vi "INI.GetSettings.vi"(8 "error in (no error)":errorcluster, 11 "INI Folder Location":path) -> (0 "error out":errorcluster, 3 "INI.Settings":T1={"Build Location"=path "C:/Simple Sequence Editor/SequenceRepo", "LoggingLocation"=path ""})   [LabVIEW 2013, in "Simple Sequence Tools - Shared.lvlib"]
uses:
  Simple Sequence Tools - Shared.lvlib
  Types/INI.Settings
  Main.Constants.vi
  <vilib>/Utility/config.llb/Read Key (Path).vi
  <vilib>/Utility/config.llb/Write Key (Path).vi
  <vilib>/Utility/config.llb/NI_LVConfig.lvlib
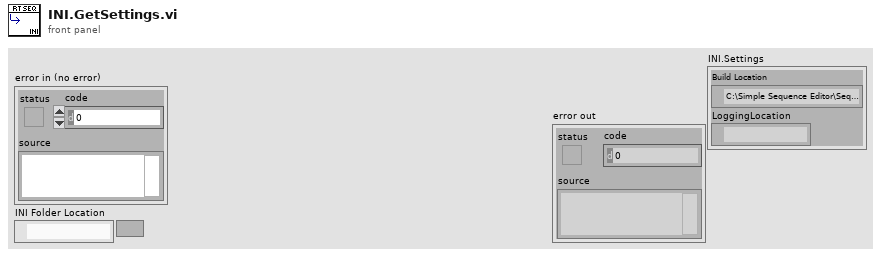
[diagram p1: front panel]
types:
  T1 = typedef "Simple Sequence Tools - Shared.lvlib/INI.Settings" = cluster{"Build Location":path, "LoggingLocation":path}
  T2 = typedef "NI_LVConfig.lvlib/Config Data RefNum.ctl" = refnum<k1>
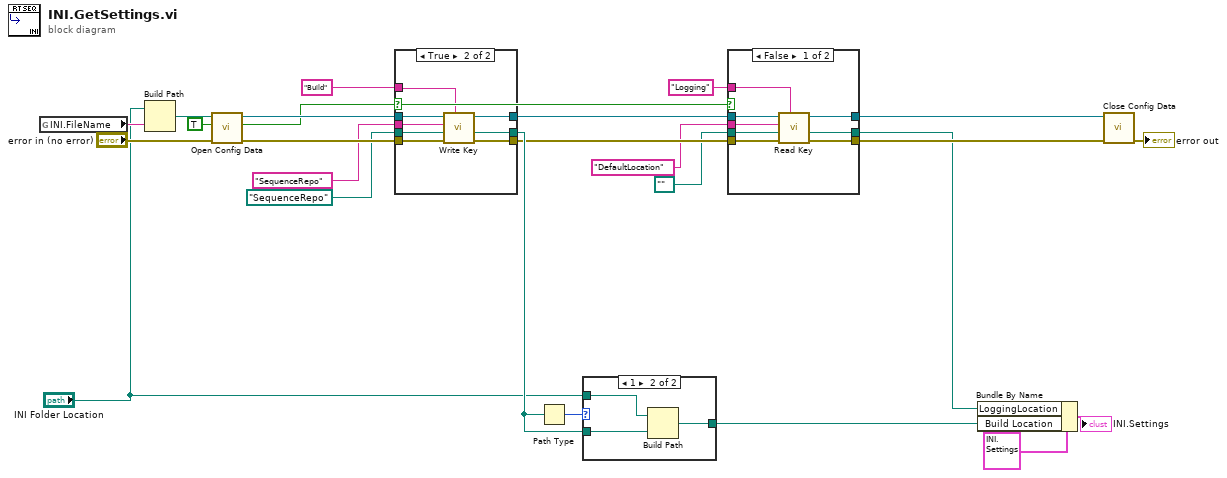
[diagram p0: block diagram]
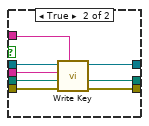
[diagram p2: hidden frame]
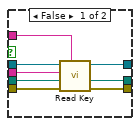
[diagram p3: hidden frame]
diagram:
  n1 = global read "Main.Constants.vi" "INI.FileName"() -> (w17:string)
  n2 = Build Path(base path="INI Folder Location", name or relative path=w17) -> (appended path=w18:path)
  n3 = call <vilib>:"Open Config Data.vi"("error in (no error)"="error in (no error)", "create file if necessary (T)"=TRUE, "configuration file path"=w18) -> ("error out"=w24:errorcluster, "file created?"=w8:bool, "refnum"=w25:T2)  [unwired: 6 in]
  n4 = case shown="True" w8 {
    tunnel: w25 -> [w33 w38]
    tunnel: w24 -> [w32 w40]
    tunnel: [w31 w36] -> w10
    tunnel: [w30 w34] -> w5
    tunnel: "Build" ("section") -> [w29 w37]
    tunnel: "SequenceRepo" ("key") -> [w28 w39]
    tunnel: path "SequenceRepo" ("default value") -> [w27 w35]
    tunnel: [w26 w35] -> w19
    frame False {
      n5 = call-poly <vilib>:"Read Key.vi"("section"=w29, "error in (no error)"=w32, "default value"=w27, "key"=w28, "refnum"=w33) -> ("error out"=w31:errorcluster, "value"=w26:path, "refnum out"=w30:T2)  [unwired: 3 in, 1 out]
    }
    frame True {
      n6 = call-poly <vilib>:"Write Key.vi"("section"=w37, "error in (no error)"=w40, "value"=w35, "key"=w39, "refnum"=w38) -> ("error out"=w36:errorcluster, "refnum out"=w34:T2)  [unwired: 4 in, 1 out]
    }
  }
  n7 = Path Type(1:w19) -> (0:w20:i16)
  n8 = case shown="1" w20 {
    tunnel: w19 -> [w41 w44]
    tunnel: [w41 w43] -> w12
    tunnel: "INI Folder Location" -> [_ w42]
    frame 0, Default {
    }
    frame 1 {
      n9 = Build Path(base path=w42, name or relative path=w44) -> (appended path=w43:path)
    }
  }
  n10 = case shown="False" w8 {
    tunnel: w5 -> [w52 w57]
    tunnel: w10 -> [w51 w59]
    tunnel: [w50 w55] -> w9
    tunnel: [w49 w53] -> w4
    tunnel: "Logging" ("section") -> [w48 w56]
    tunnel: "DefaultLocation" ("key") -> [w47 w58]
    tunnel: path "" ("default value") -> [w46 w54]
    tunnel: [w45 w54] -> w2
    frame False {
      n11 = call-poly <vilib>:"Read Key.vi"("section"=w48, "error in (no error)"=w51, "default value"=w46, "key"=w47, "refnum"=w52) -> ("error out"=w50:errorcluster, "value"=w45:path, "refnum out"=w49:T2)  [unwired: 3 in, 1 out]
    }
    frame True {
      n12 = call-poly <vilib>:"Write Key.vi"("section"=w56, "error in (no error)"=w59, "value"=w54, "key"=w58, "refnum"=w57) -> ("error out"=w55:errorcluster, "refnum out"=w53:T2)  [unwired: 4 in, 1 out]
    }
  }
  n13 = Bundle By Name(cluster=T1 {"Build Location"=path "C:/Simple Sequence Editor/SequenceRepo", "LoggingLocation"=path ""}, "LoggingLocation"=w2, "Build Location"=w12) -> (→"INI.Settings":T1)
  n14 = call <vilib>:"Close Config Data.vi"("error in (no error)"=w9, "refnum"=w4) -> ("error out"=→"error out":errorcluster)  [unwired: 8 in, 1 out]
